vi "Scan read phase v_2 axis (SubVI).vi"(6 "Y":i32, 7 "General VI":refnum<vi>, 8 "error in (no error)":errorcluster, 9 "Y_size":i32, 10 "X_size":i32, 11 "VISA Refnum in":refnum<visa-resource-name>) -> (0 "error out":errorcluster, 1 "X":i32, 2 "value":dbl[](array[numeric]), 3 "VISA Refnum out":refnum<visa-resource-name>)   [LabVIEW 2018]
uses:
  GlobalStop.vi
  <vilib>/regexp/Match Regular Expression.xnode
panel:
  out "succes, %":i32
  out "err":errorcluster
  out "POS":i32[](array[numeric])
  out "error":errorcluster
  out "str_array":string[][](array[string])
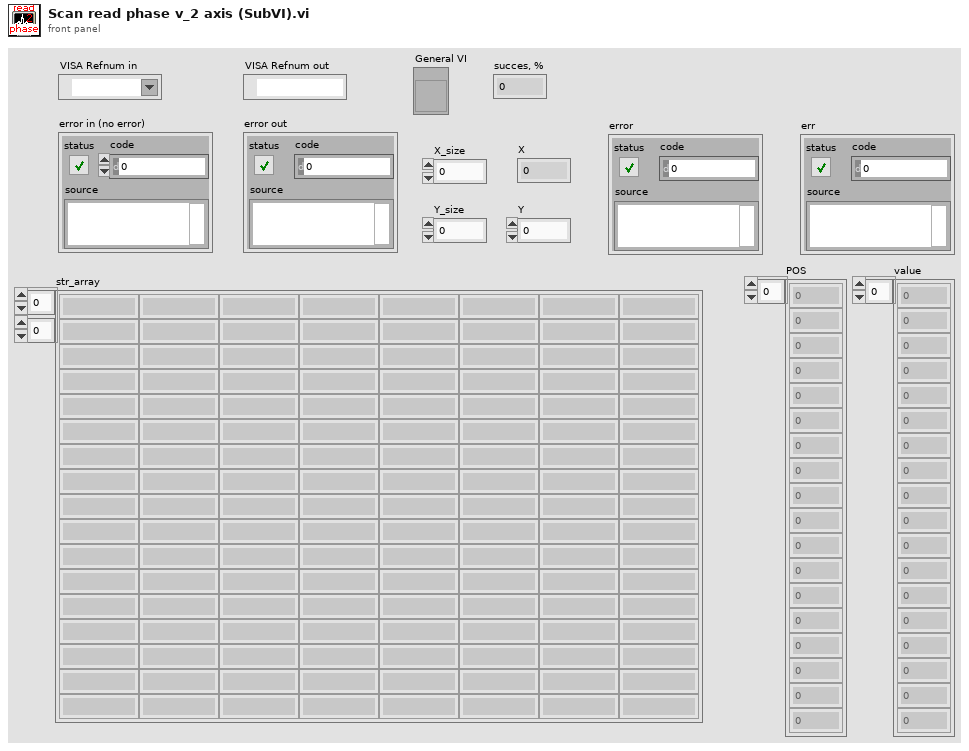
[diagram p1: front panel]
types:
  T1 = enum32{"Invalid", "Standard", "Closed", "Hidden", "Minimized", "Maximized"}
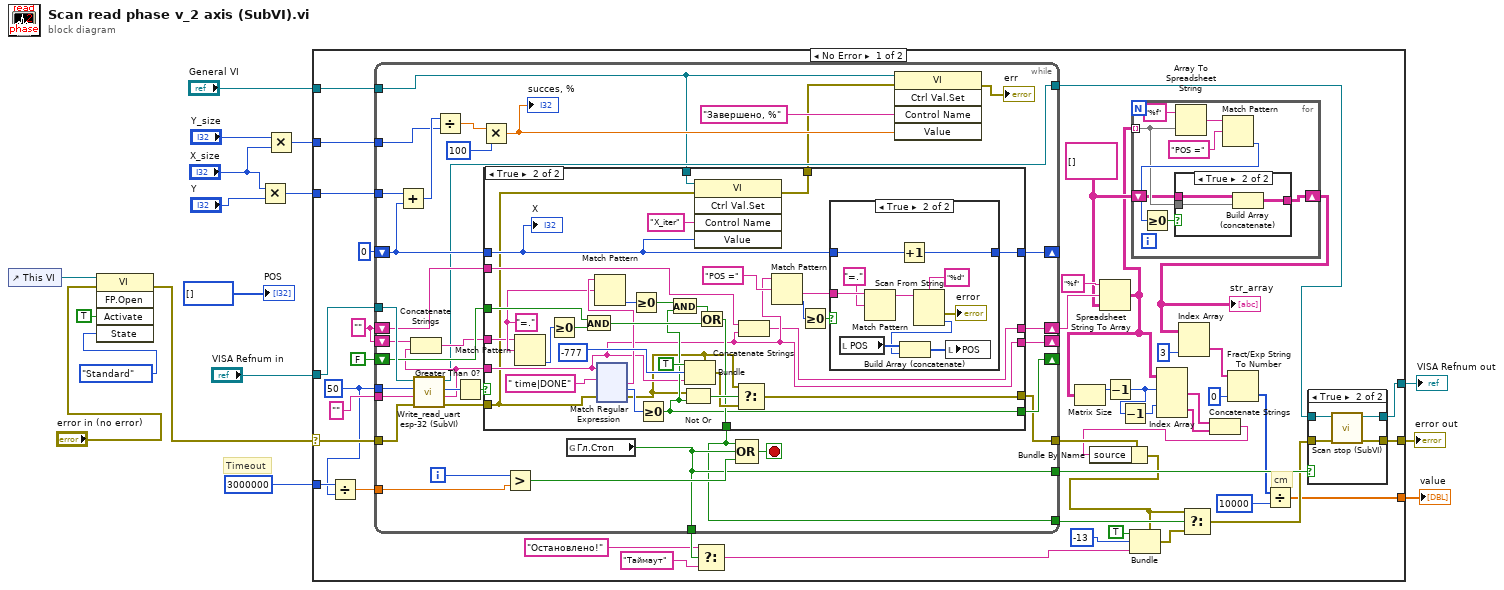
[diagram p0: block diagram]
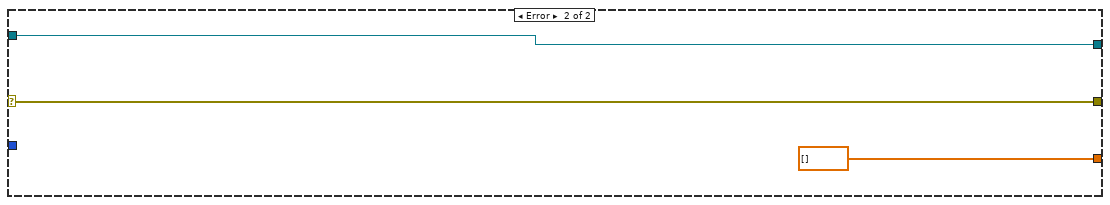
[diagram p6: hidden frame]
diagram:
  # "Timeout"
  n1 = control-ref of="This VI"() -> (w2:refnum<vi>)
  n2 = invoke class="VI" method="FP.Open"(reference=w2, error in="error in (no error)", "Activate"=TRUE, "State"=T1."Standard") -> (error out=w1:errorcluster)  [unwired: 1 in, 4 out]
  n3 = Multiply(x="X_size", y="Y") -> (x*y=w6:i32)
  n4 = Multiply(x="Y_size", y="X_size") -> (x*y=w9:i32)
  n5 = case shown="No Error" w1 {
    selector: w1 -> [w59 w279]
    tunnel: "VISA Refnum in" -> [w61 w280]
    tunnel: [w52 w280] -> w13
    tunnel: [w29 dbl[] []] -> w15
    tunnel: [w50 w279] -> w14
    tunnel: 3000000 -> [w47 _]
    tunnel: "General VI" -> [w26 _]
    tunnel: w9 -> [w24 _]
    tunnel: w6 -> [w23 _]
    frame No Error {
      w20 = string[][] [] ("Array")
      w30 = ""
      w46 = u32 50 ("milliseconds to wait")
      # "cm"
      n6 = Divide(x=w47, y=w46) -> (x/y=w45:dbl)
      n7 = while {
        tunnel: w46 -> [w114]
        tunnel: "" ("write buffer") -> [w111]
        tunnel: [w102] -> w51
        tunnel: [w103] -> w56
        tunnel: [w103] -> w49
        tunnel: w45 -> [w105]
        shift-right: [w109] -> w42
        shift-left: w30 -> [w108]
        shift-right: [w99] -> _
        shift-left: FALSE -> [w98]
        shift-right: [w97] -> _
        shift-left: w30 -> [w96]
        tunnel: w61 -> [w113]
        tunnel: w26 -> [w81]
        shift-right: [w92] -> _
        shift-left: 0 -> [w90]
        tunnel: w24 -> [w88]
        tunnel: w23 -> [w91]
        tunnel: [w82] -> w22
        tunnel: w59 -> [w112]
        tunnel: [w93] -> w39
        i -> [w106]
        stop <- w107 stop-if-true
        n8 = Add(x=w91, y=w90) -> (x+y=w89:i32)
        n9 = call "Write_read_uart esp-32 (SubVI).vi"("error in (no error)"=w112, "write buffer"=w111, "milliseconds to wait"=w114, "VISA Refnum in"=w113) -> ("error out 4"=w101:errorcluster, "read buffer"=w94:string, "read bite"=w110:u32, "VISA resource name out"=w82:refnum<visa-resource-name>)
        n10 = Concatenate Strings(w96, w94) -> (w95:string)
        n11 = Divide(x=w89, y=w88) -> (x/y=w87:dbl)
        n12 = Greater Than 0?(x=w110) -> (x > 0?=w100:bool)
        n13 = Multiply(x=w87, y=100) -> (x*y=w85:dbl)
        "succes, %" <- w85
        n14 = case shown="True" w100 {
          selector: w100 -> [w119 _]
          tunnel: [w118 w130] -> w109
          tunnel: w108 -> [w118 w133]
          tunnel: [w119 w142] -> w102
          tunnel: w94 -> [w117 w131]
          tunnel: w101 -> [w115 w120]
          tunnel: [w115 w150] -> w93
          tunnel: [w119 w135] -> w99
          tunnel: w98 -> [_ w143]
          tunnel: [w117 w131] -> w97
          tunnel: w95 -> [_ w134]
          tunnel: w90 -> [w116 w124]
          tunnel: [w116 w126] -> w92
          tunnel: w81 -> [_ w122]
          tunnel: [w115 w121] -> w80
          frame False {
          }
          frame True {
            w139 = "=." ("f")
            n15 = Match Pattern(string=w134, regular expression=w139) -> (offset past match=w145:i32)  [unwired: 1 in, 3 out]
            n16 = Greater Or Equal To 0?(x=w145) -> (x >= 0?=w144:bool)
            n17 = And(x=w143, y=w144) -> (x .and. y?=w141:bool)
            n18 = xnode "Match Regular Expression"("input string"=w131, "regular expression"=" time|DONE", "error in"=w120) -> ("after match"=w140:string, "offset past match"=w151:i32, "error out"=w123:errorcluster)  [unwired: 3 in, 2 out]
            n19 = Match Pattern(string=w140, regular expression=w139) -> (offset past match=w138:i32)  [unwired: 1 in, 3 out]
            n20 = Greater Or Equal To 0?(x=w138) -> (x >= 0?=w137:bool)
            n21 = Greater Or Equal To 0?(x=w151) -> (x >= 0?=w135:bool)
            n22 = And(x=w137, y=w135) -> (x .and. y?=w136:bool)
            n23 = Not Or(1:w135, 2:w123) -> (0:w147:bool)
            n24 = Bundle(cluster=w123, "status"=TRUE, "code"=-777, "source"=w131) -> (w146:errorcluster)
            n25 = invoke class="VI" method="Ctrl Val.Set"(reference=w122, error in=w120, "Control Name"="X_iter", "Value"=w124) -> (error out=w121:errorcluster)  [unwired: 1 in, 4 out]
            n26 = Or(x=w136, y=w141) -> (x .or. y?=w142:bool)
            n27 = Select(t=w123, s=w147, f=w146) -> (s? t:f=w150:errorcluster)
            n28 = Concatenate Strings(w133, w131) -> (w130:string)
            n29 = Match Pattern(string=w131, regular expression="POS =") -> (after substring=w127:string, offset past match=w129:i32)  [unwired: 1 in, 2 out]
            n30 = Greater Or Equal To 0?(x=w129) -> (x >= 0?=w128:bool)
            n31 = case shown="True" w128 {
              tunnel: w127 -> [_ w163]
              tunnel: w124 -> [w153 w155]
              tunnel: [w153 w154] -> w126
              frame False {
              }
              frame True {
                n32 = local read "POS"() -> (w158:i32[])
                n33 = Match Pattern(string=w163, regular expression="=.") -> (before substring=w161:string)  [unwired: 1 in, 3 out]
                n34 = Increment(x=w155) -> (x+1=w154:i32)
                n35 = Scan From String(format string="%d", input string=w161) -> (error out=→"error":errorcluster, output 1=w157:i32)  [unwired: 3 in, 2 out]
                n36 = Build Array (concatenate)(w158, w157) -> (w156:i32[])
                n37 = local write "POS"(w156) -> ()
              }
            }
            "X" <- w124
          }
        }
        n38 = Greater?(x=w106, y=w105) -> (0:w104:bool)
        n39 = global read "GlobalStop.vi" "Гл.Стоп"() -> (w103:bool)
        n40 = Compound Arithmetic op=OR(w102, w103, w104) -> (w107:bool)
        n41 = invoke class="VI" method="Ctrl Val.Set"(reference=w81, error in=w80, "Control Name"="Завершено, %", "Value"=w85) -> (error out=→"err":errorcluster)  [unwired: 1 in, 4 out]
      }
      n42 = Select(t="Остановлено!" ("regular expression"), s=w56, f="Таймаут") -> (s? t:f=w55:string)
      n43 = Spreadsheet String To Array(format string="%f", spreadsheet string=w42, array type (2D Dbl)=w20) -> (array=w18:string[][])  [unwired: 1 in]
      n44 = Matrix Size(0:w18) -> (1:w38:i32)  [unwired: 1 out]
      n45 = Decrement(x=w38) -> (x-1=w37:i32)
      n46 = Decrement(x=w37) -> (x-1=w36:i32)
      n47 = for {
        tunnel: w18 -> [w65] mode=indexing
        shift-right: [w64] -> w21
        shift-left: w20 -> [w63]
        n48 = Array To Spreadsheet String(array=w65, 3:"%f" ("format string")) -> (spreadsheet string=w69:string)  [unwired: 1 in]
        n49 = Match Pattern(string=w69, regular expression="POS =") -> (offset past match=w67:i32)  [unwired: 1 in, 3 out]
        n50 = Greater Or Equal To 0?(x=w67) -> (x >= 0?=w66:bool)
        n51 = case shown="True" w66 {
          tunnel: w65 -> [_ w73]
          tunnel: [w70 w72] -> w64
          tunnel: w63 -> [w70 w71]
          frame False {
          }
          frame True {
            n52 = Build Array (concatenate)(w71, w73) -> (w72:string[][])
          }
        }
      }
      "str_array" <- w21
      n53 = Index Array(array=w18, index (row) #1=w37, index (row) #2=w36) -> (element #1=w35:string[], element #2=w34:string[])  [unwired: 2 in]
      n54 = Index Array(array=w21, index (col)=3 ("index (row)")) -> (element=w19:string[])  [unwired: 1 in]
      n55 = Concatenate Strings(w35, w34) -> (w33:string)
      n56 = Bundle By Name(cluster=w39, "source"=w33) -> (w32:errorcluster)
      n57 = Bundle(cluster=w32, "status"=TRUE, "code"=-13, "source"=w55) -> (w48:errorcluster)
      n58 = Select(t=w32, s=w51, f=w48) -> (s? t:f=w40:errorcluster)
      n59 = Fract/Exp String To Number(string=w19, default (0 dbl)=i16 0 ("default (0 DBL)")) -> (number=w28:i16[])  [unwired: 3 out]
      n60 = Divide(x=w28, y=10000) -> (x/y=w29:dbl[])
      n61 = case shown="True" w49 {
        tunnel: w22 -> [w74 w79]
        tunnel: [w74 w78] -> w52
        tunnel: w40 -> [w75 w76]
        tunnel: [w75 w77] -> w50
        frame False {
        }
        frame True {
          n62 = call "Scan stop (SubVI).vi"("error in"=w76, "VISA Refnum in"=w79) -> ("error out"=w77:errorcluster, "VISA Refnum out"=w78:refnum<visa-resource-name>)  [unwired: 8 in]
        }
      }
    }
    frame Error {
    }
  }
  "VISA Refnum out" <- w13
  "error out" <- w14
  "value" <- w15
  "POS" <- i32[] [] ("POS")
